vi "TestStand - GetProjectBuildSpecs.vi"(11 "Project Path":path) -> (3 "PPL Build Specs":string[](array[string]))   [LabVIEW 2014]
panel:
  out "All Build Specs":string[](array[string])
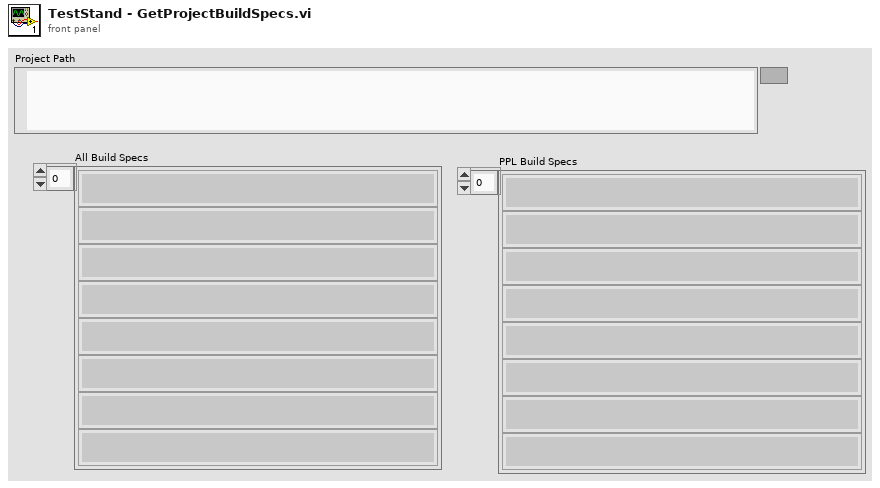
[diagram p1: front panel]
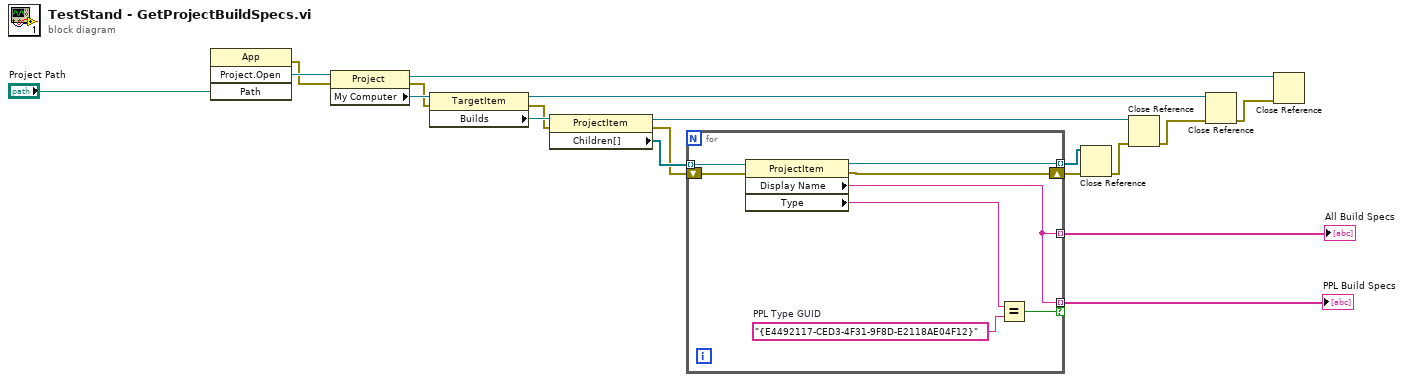
[diagram p0: block diagram]
diagram:
  n1 = invoke class="App" method="Project.Open"("Path"="Project Path") -> (error out=w9:errorcluster, "Project:Open"=w18:refnum<vi>)  [unwired: 3 in, 2 out]
  n2 = property class="Project"(reference=w18, error in=w9) -> (reference out=w4:refnum<vi>, error out=w10:errorcluster, "My Computer"=w17:refnum<vi>)
  n3 = property class="TargetItem"(reference=w17, error in=w10) -> (reference out=w5:refnum<vi>, error out=w11:errorcluster, "Builds"=w16:refnum<vi>)
  n4 = property class="ProjectItem"(reference=w16, error in=w11) -> (reference out=w6:refnum<vi>, error out=w12:errorcluster, "Children[]"=w15:refnum<vi>[])
  n5 = for {
    tunnel: w15 -> [w27] mode=indexing
    tunnel: [w24] -> w14 mode=indexing
    tunnel: [w24] -> w13 mode=indexing if=w23
    tunnel: [w22] -> w8 mode=indexing
    shift-right: [w21] -> w7
    shift-left: w12 -> [w20]
    w26 = "{E4492117-CED3-4F31-9F8D-E2118AE04F12}"  # PPL Type GUID
    n6 = property class="ProjectItem"(reference=w27, error in=w20) -> (reference out=w22:refnum<vi>, error out=w21:errorcluster, "Display Name"=w24:string, "Type"=w25:string)
    n7 = Equal?(x=w25, y=w26) -> (x = y?=w23:bool)
  }
  "All Build Specs" <- w14
  "PPL Build Specs" <- w13
  n8 = Close Reference(reference=w8, error in (no error)=w7) -> (error out=w3:errorcluster)
  n9 = Close Reference(reference=w6, error in (no error)=w3) -> (error out=w2:errorcluster)
  n10 = Close Reference(reference=w5, error in (no error)=w2) -> (error out=w1:errorcluster)
  n11 = Close Reference(reference=w4, error in (no error)=w1) -> ()  [unwired: 1 out]
